vi "Atitude Control Test.vi"() -> ()   [LabVIEW 2013]
uses:
  lv-attitudecontrol.lvlib
panel:
  in  "Attitude Indicator":refnum<vi>(3d-picture)
  in  "stop":bool
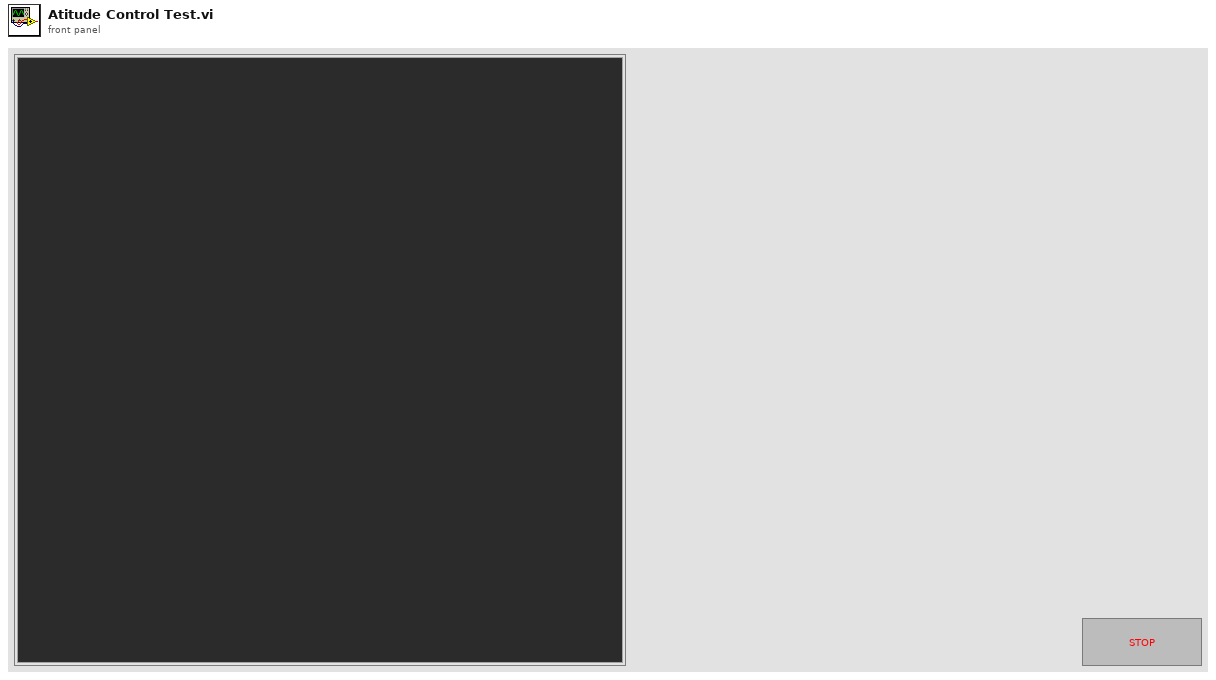
[diagram p1: front panel]
types:
  T1 = typedef "lv-attitudecontrol.lvlib/AttitudeHandle.ctl" = cluster{"First Scene Object":refnum<vi>, "Drum":refnum<vi>, "Window":refnum<vi>, "Dial":refnum<vi>, "Scene Graph":refnum<vi>, "Last Drum Pitch":dbl, "Last Drum Roll ":dbl, "Last Dial Roll":dbl}
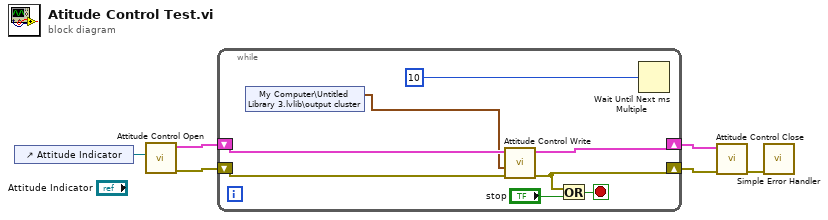
[diagram p0: block diagram]
diagram:
  n1 = control-ref of="Attitude Indicator"() -> (w4:refnum<vi>)
  n2 = call "Attitude Control Open.vi"("Scene Graph"=w4) -> ("error out"=w5:errorcluster, "Attitude Control Handle"=w6:T1)  [unwired: 9 in]
  n3 = while {
    shift-right: [w9] -> w2
    shift-left: w6 -> [w14]
    shift-right: [w10] -> w3
    shift-left: w5 -> [w13]
    stop <- w11 stop-if-true
    n4 = shared-variable "My Computer\\Untitled Library 3.lvlib\\output cluster"() -> (w7:cluster{dbl, dbl, dbl})  [unwired: 1 in, 1 out]
    n5 = call "Attitude Control Write.vi"("error in (no error)"=w13, "Cluster"=w7, "Attitude Control Handle In"=w14) -> ("error out"=w10:errorcluster, "Attitude Control Handle Out"=w9:T1)  [unwired: 7 in]
    n6 = Or(x=w10, y="stop") -> (x .or. y?=w11:bool)
    n7 = Wait Until Next ms Multiple(millisecond multiple=u32 10) -> ()  [unwired: 1 out]
  }
  n8 = call "Attitude Control Close.vi"("error in (no error)"=w3, "Attitude Control Handle"=w2) -> ("error out"=w1:errorcluster)  [unwired: 9 in]
  n9 = call <vilib>:"Simple Error Handler.vi"("error in (no error)"=w1) -> ()  [unwired: 4 in, 5 out]
